vi "Configure Output Enabled.vi"(6 "Settle (1mS)":u32=1, 8 "error in (no error)":errorcluster, 10 "Enable Output (F: Off)":bool, 11 "VISA resource name":refnum<visa-resource-name>) -> (0 "error out":errorcluster, 3 "VISA resource name out":refnum<visa-resource-name>)   [LabVIEW 2018, in "TDK-Lambda Z.lvlib"]
doc: "Sets the power supply output On or Off. No other settings change.\nIf \"Output On\" is set False, the output will be turned Off.\n\nNote: This VI will wait for \"Settle\" milliseconds after setting the output. If unwired, there will be no delay"
uses:
  TDK-Lambda Z.lvlib
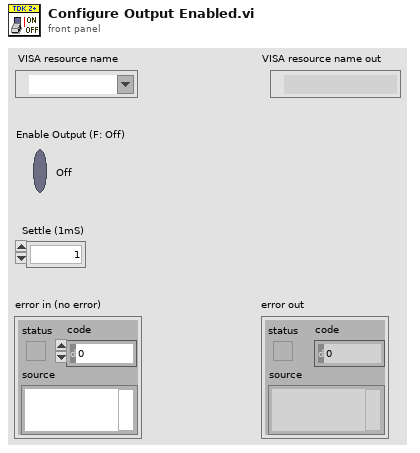
[diagram p1: front panel]
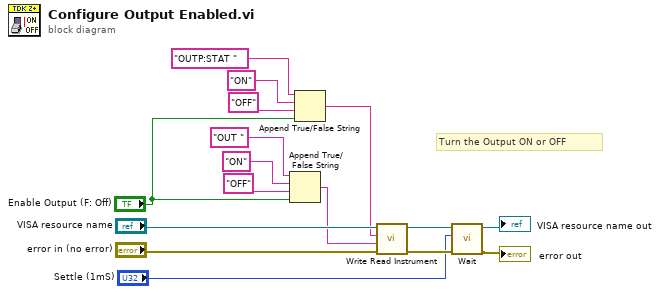
[diagram p0: block diagram]
diagram:
  # "Turn the Output ON or OFF"
  n1 = Append True/False String(1:"Enable Output (F: Off)", 2:"OFF" ("format string"), 3:"ON" ("format string"), 4:"OUT " ("format string")) -> (0:w2:string)
  n2 = Append True/False String(1:"Enable Output (F: Off)", 2:"OFF" ("format string"), 3:"ON" ("format string"), 4:"OUTP:STAT " ("format string")) -> (0:w8:string)
  n3 = call "Write Read Instrument.vi"("error in (no error)"="error in (no error)", "GEN  Write Command/Query"=w2, "SCPI  Write Command/Query"=w8, "VISA resource name"="VISA resource name") -> ("error out"=w13:errorcluster, "VISA resource name out"=w14:refnum<visa-resource-name>)  [unwired: 5 in, 1 out]
  n4 = call "Wait.vi"("error in (no error)"=w13, "Wait (1mS)"="Settle (1mS)", "VISA resource name"=w14) -> ("error out"=→"error out":errorcluster, "VISA resource name out"=→"VISA resource name out":refnum<visa-resource-name>)  [unwired: 7 in]
